vi "Request Data.vi"(11 "Address counter":u32) -> (3 "Address counter output":u32)   [LabVIEW 2015]
uses:
  <vilib>/rvi/Memory/Memory_Emulation/niFpgaMemoryEmulationDramWriteAndRequestData.vi
  <vilib>/rvi/Memory/Memory_Emulation/niFpgaMemoryFastEmulationDramWriteAndRequestData.vi
  <vilib>/rvi/DataTransferAndStorage/Container/Common/niFpgaContainerGetUniqueNameForEmu.vi
  <vilib>/rvi/Memory/Memory_Emulation/niFpgaMemoryEmulationCacheClearOnFirstRun.vi
  <vilib>/rvi/Memory/Memory_Emulation/nirvimemoryEmulationManagerCache_MakeExclusive.vi
  <vilib>/rvi/Memory/Memory_Emulation/nirvimemoryEmulationManagerCache_GetValue.vi
  <vilib>/rvi/Memory/Memory_Emulation/nirvimemoryEmulationManagerCache_InsertValue.vi
  <vilib>/Utility/error.llb/Clear Errors.vi
  <vilib>/rvi/Memory/Memory_Emulation/nirvimemoryEmulationManagerCache_ReleaseExclusive.vi
  <vilib>/rvi/Memory/Memory_Emulation/niFpgaMemoryEmulationDramWriteAndRequestDataApplyByteEnables.vi
  <vilib>/rvi/Memory/Memory_Emulation/nirvimemoryEmulationManagerCache_SetValue.vi
  <vilib>/rvi/DataTransferAndStorage/Container/XNode/niFpgaContainer.xnode
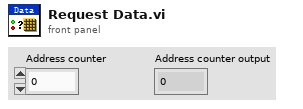
[diagram p1: front panel]
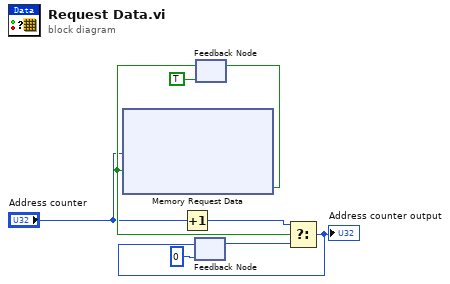
[diagram p0: block diagram]
diagram:
  n1 = Increment(x="Address counter") -> (x+1=w6:u32)
  n2 = feedback #1(u32 0) -> (w4:u32)
  n3 = feedback #2(TRUE ("Ready for Input")) -> (w3:bool)
  n4 = xnode ("Memory Request Data")("地址"="Address counter", "输入有效"=w3) -> ("输入就绪"=w1:bool)  [unwired: 1 in, 1 out]
  n5 = feedback-in #2(w1) -> ()
  n6 = Select(t=w6, s=w3, f=w4) -> (s? t:f=w5:u32)
  "Address counter output" <- w5
  n7 = feedback-in #1(w5) -> ()
